vi "Do_Every_minute.vi"(1 "Ch Names":string[](array[string]), 2 "Values":dbl[](array[numeric]) format="%.2f") -> ()   [LabVIEW 2014]
uses:
  Do_Every_5mins.ctl
  Anemometry/Anemometry Sub Vis/Controls/In_Range.ctl
  ADAM Client/Sub VIs/ADAM Controls/Traverse_Level_State.ctl
  ADAM Client/Sub VIs/ADAM Controls/Valco_valve_ph.ctl
  <vilib>/Analysis/baseanly.llb/Mean (DBL).vi
  ADAM_Global.vi
  <vilib>/Analysis/NI_AALBase.lvlib
panel:
  in  "Disable Sending email to estates regarding Chilled water Temp":bool=TRUE
  in  "Max K Factor":dbl=2.7
  out "Case":T1
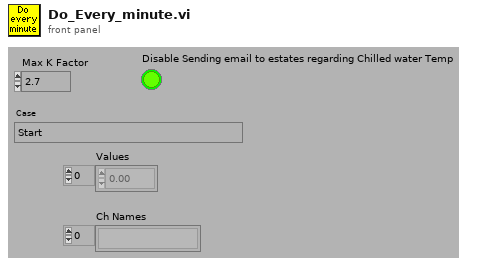
[diagram p1: front panel]
types:
  T1 = typedef "Do_Every_5mins.ctl" = enum16{"Start", "Update EnFlo Tunnel Speed Tweak", "Are EnFlo Tun Fan Bearings too Hot?", "Check EnFlo tweak factor?", "Are Inlet Screens Blocked?", "Tweak demanded chilled water temp", "Is Dew point meter Alive?", "Condensation Occurring", "Condensation Alert", "More checks", "Set FFID Valve to Measure", "End"}
  T2 = typedef "In_Range.ctl" = enum16{"%", "±", "% & ±"}
  T3 = typedef "Traverse_Level_State.ctl" = enum16{"Running", "Complete"}
  T4 = typedef "Client_State_Cluster.ctl" = cluster{"Client Name":string, "Traverse level State":T3, "People to Email":string[], "Next Contact Time":dbl}
  T5 = typedef "Valco_valve_ph.ctl" = u16
  T6 = cluster{"second":i32, "minute":i32, "hour":i32, "day of month":i32, "month":i32, "year":i32, "day of week":i32, "day of year":i32, "is DST":i32}
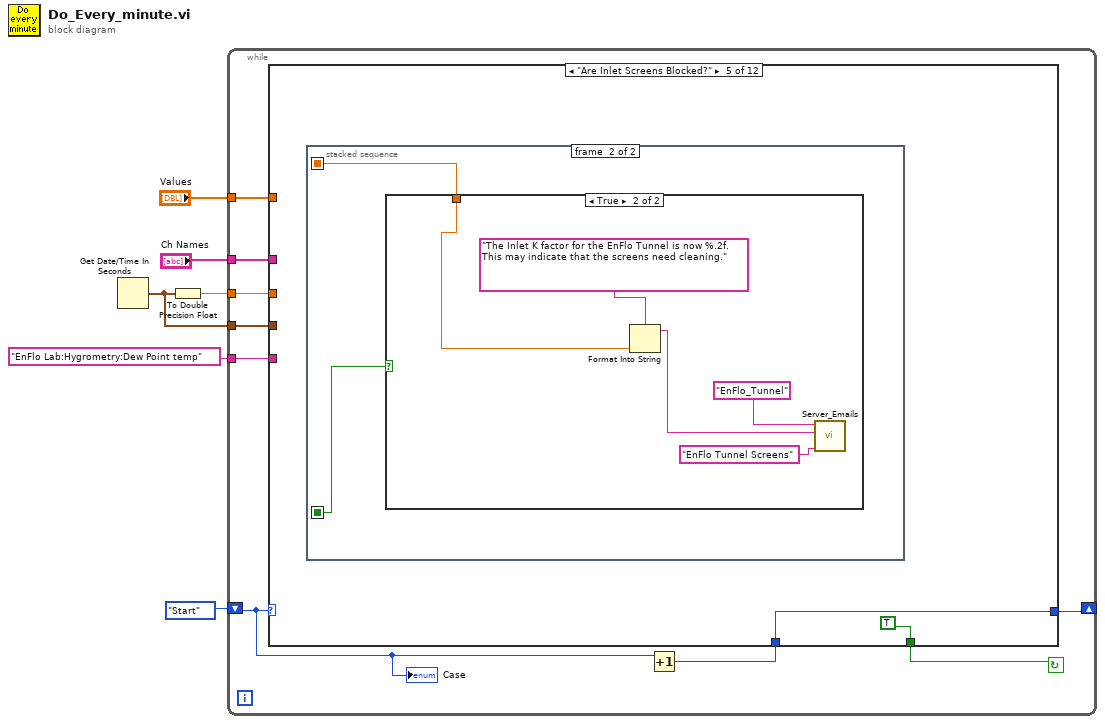
[diagram p0: block diagram]
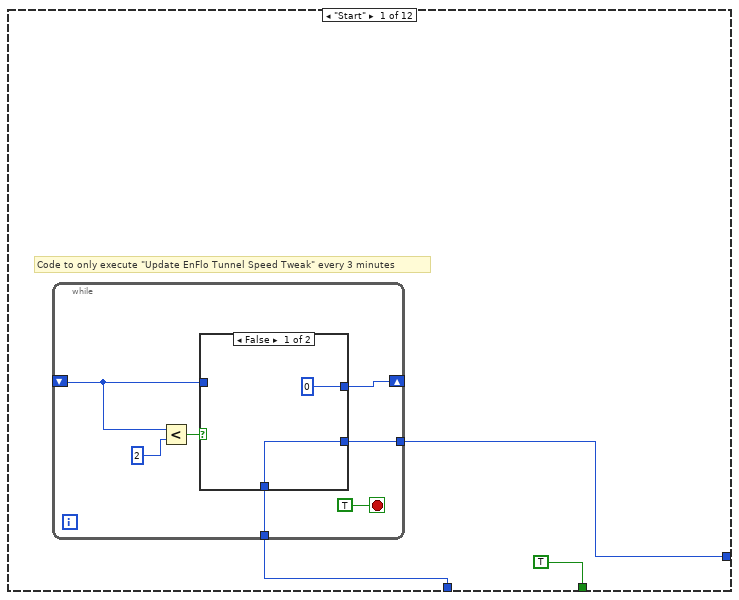
[diagram p2: hidden frame]
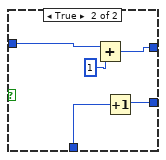
[diagram p3: hidden frame]
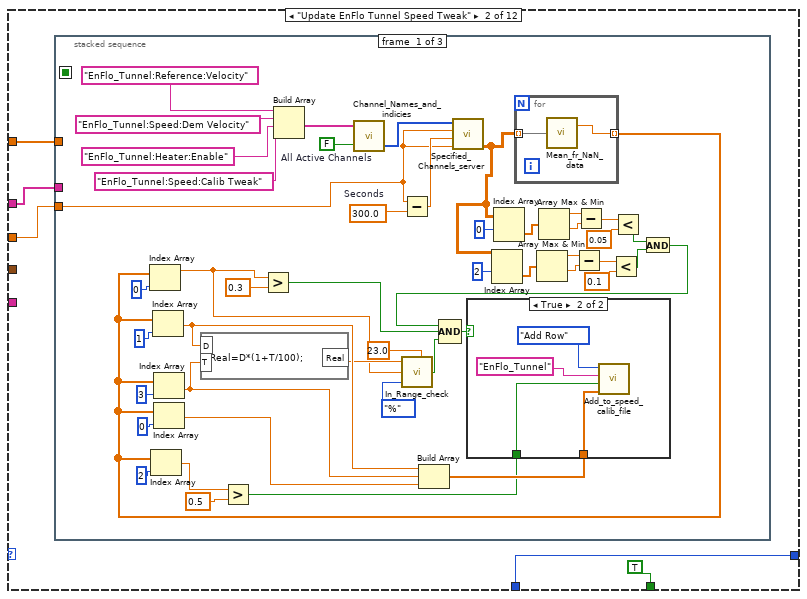
[diagram p4: hidden frame]
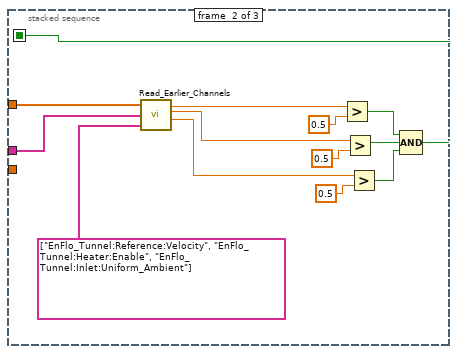
[diagram p6: hidden frame]
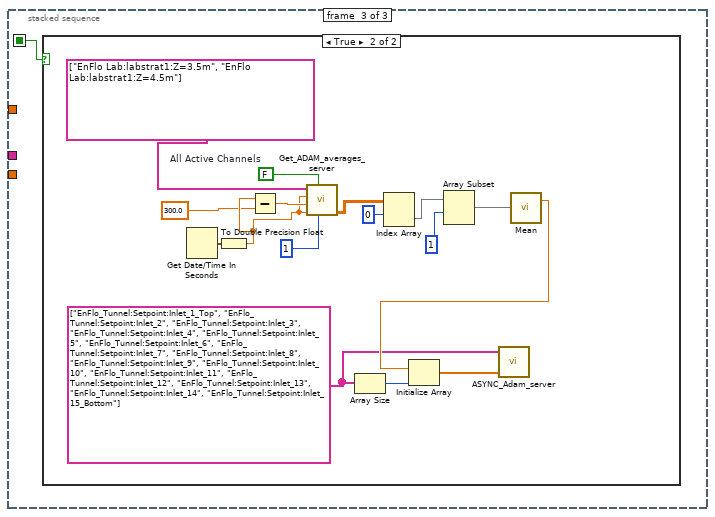
[diagram p7: hidden frame]
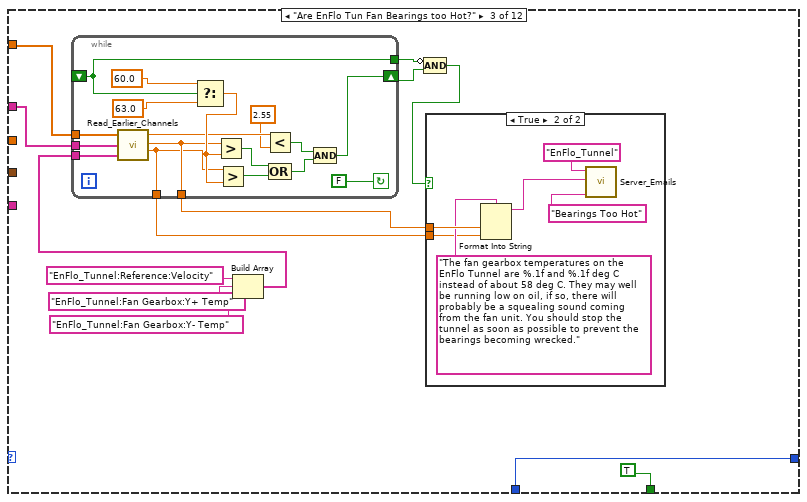
[diagram p9: hidden frame]
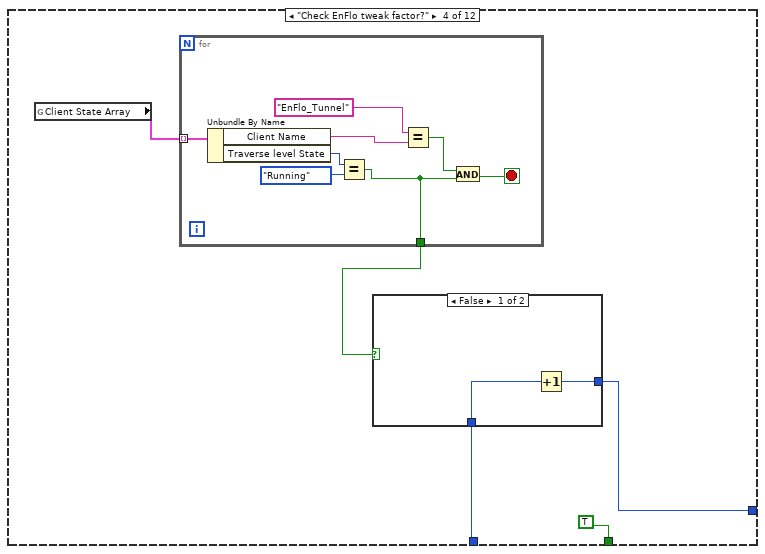
[diagram p11: hidden frame]
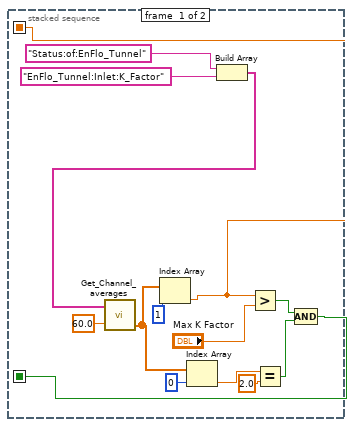
[diagram p13: hidden frame]
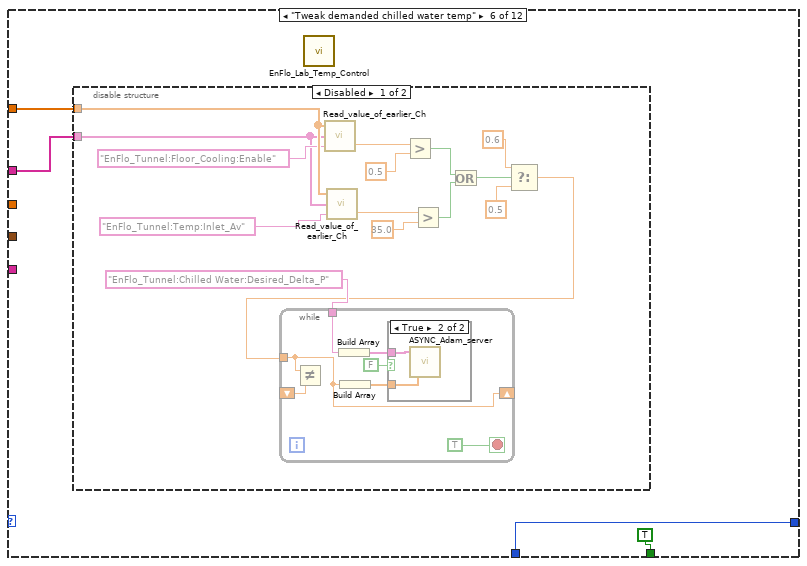
[diagram p15: hidden frame]
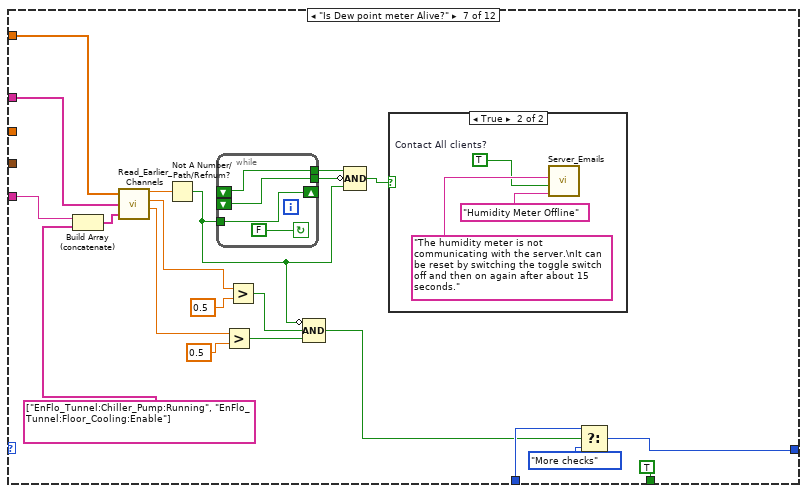
[diagram p18: hidden frame]
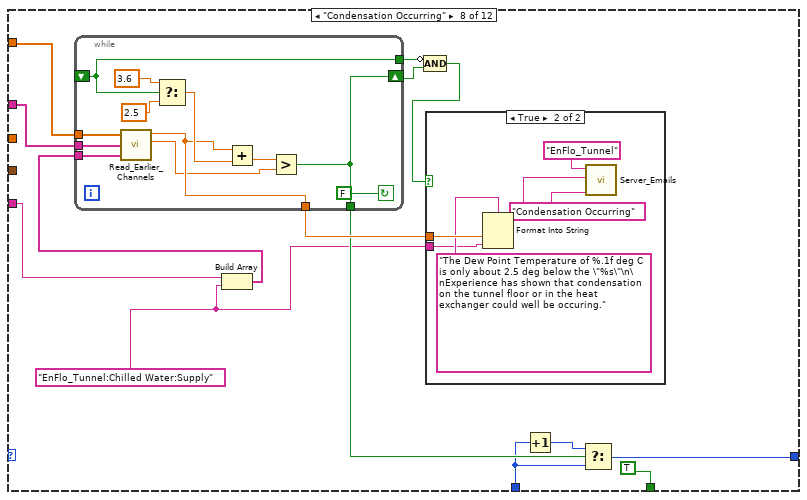
[diagram p20: hidden frame]
diagram:
  n1 = Get Date/Time In Seconds() -> (seconds since 1Jan1904=w1:timestamp)
  n2 = To Double Precision Float(number=w1) -> (double precision float=w2:dbl)
  n3 = while {
    tunnel: "EnFlo Lab:Hygrometry:Dew Point temp" -> [w9]
    tunnel: "Values" -> [w13]
    tunnel: "Ch Names" -> [w14]
    shift-left: Do_Every_5mins."Start" ("Case") -> [w10]
    shift-right: [w11] -> _
    tunnel: w2 -> [w8]
    tunnel: w1 -> [w7]
    stop <- w15 continue-if-true
    n4 = Increment(x=w10) -> (x+1=w12:T1)
    n5 = case shown="\"Are Inlet Screens Blocked?\"" w10 {
      tunnel: [TRUE TRUE TRUE TRUE TRUE TRUE TRUE TRUE TRUE TRUE TRUE FALSE] -> w15
      tunnel: w14 -> [_ w34 w130 _ _ w196 w240 w263 w290 w333 w342 w376]
      tunnel: w13 -> [_ w33 w131 _ _ w197 w241 w264 w291 w334 w341 w375]
      tunnel: w12 -> [w16 w37 w121 w159 w173 w199 w234 w254 w293 w331 w360 w379]
      tunnel: [w17 w37 w121 w158 w173 w199 w244 w255 w293 w330 w360 w379] -> w11
      tunnel: w9 -> [_ _ _ _ _ _ w239 w257 w284 _ _ _]
      tunnel: w8 -> [_ w35 _ _ _ _ _ _ _ _ w359 w374]
      tunnel: w7 -> [_ _ _ _ _ _ _ _ _ _ _ w377]
      frame "Start" {
        # "Code to only execute \"Update EnFlo Tunnel Speed Tweak\" every 3 minutes"
        n6 = while {
          shift-right: [w22] -> _
          shift-left: _ -> [w19]
          tunnel: [w21] -> w17
          tunnel: w16 -> [w20]
          stop <- TRUE stop-if-true
          n7 = Less?(x=w19, y=2) -> (x < y?=w23:bool)
          n8 = case shown="False" w23 {
            tunnel: [0 w30] -> w22
            tunnel: [w26 w28] -> w21
            tunnel: w20 -> [w26 w29]
            tunnel: w19 -> [_ w31]
            frame False {
            }
            frame True {
              n9 = Add(x=w31, y=1) -> (x+y=w30:i32)
              n10 = Increment(x=w29) -> (x+1=w28:T1)
            }
          }
        }
      }
      frame "Update EnFlo Tunnel Speed Tweak" {
        n11 = stacked-sequence {
          seq-local: [_ w91 _] -> [_ _ w104]
          tunnel: w35 -> [w38 _ _]
          tunnel: w34 -> [_ w103 _]
          tunnel: w33 -> [_ w102 _]
          frame #0 {
            w69 = 300.0  # Seconds
            w71 = FALSE  # All Active Channels
            n12 = Build Array("EnFlo_Tunnel:Reference:Velocity", "EnFlo_Tunnel:Speed:Dem Velocity", "EnFlo_Tunnel:Heater:Enable", "EnFlo_Tunnel:Speed:Calib Tweak") -> (w68:string[])
            n13 = call "Channel_Names_and_indicies.vi"("All Active Channels"=w71, "Desired Ch Names"=w68) -> ("Indicies"=w70:i32[])  [unwired: 1 out]
            n14 = Subtract(x=w38, y=w69) -> (x-y=w67:dbl)
            n15 = call "Specified_Channels_server.vi"("End time"=w38, "Start time"=w67, "Clients time"=w38, "Requested channels"=w70) -> ("Output array"=w49:dbl[][])  [unwired: 1 in, 4 out]
            n16 = Index Array(array=w49, index (row)=2 ("Index")) -> (element=w51:dbl[])  [unwired: 1 in]
            n17 = Index Array(array=w49, index (row)=0 ("Index")) -> (element=w65:dbl[])  [unwired: 1 in]
            n18 = for {
              tunnel: w49 -> [w86] mode=indexing
              tunnel: [w85] -> w58 mode=indexing
              n19 = call "Mean_fr_NaN_data.vi"("Data"=w86) -> ("Mean value"=w85:dbl)  [unwired: 1 out]
            }
            n20 = Index Array(array=w58, index=0) -> (element=w42:dbl)
            n21 = Index Array(array=w58, index=2) -> (element=w76:dbl)
            n22 = Index Array(array=w58, index=1) -> (element=w44:dbl)
            n23 = Index Array(array=w58, index=3) -> (element=w45:dbl)
            n24 = Index Array(array=w58, index=0) -> (element=w56:dbl)
            n25 = formula code="Real=D*(1+T/100);"("D"=w44, "T"=w45) -> ("Real"=w43:dbl)
            n26 = Greater?(x=w76, y=0.5) -> (0:w57:bool)
            n27 = Greater?(x=w42, y=0.3) -> (0:w74:bool)
            n28 = call "In_Range_check.vi"("%"=23.0, "Mode"=In_Range."%", "Value"=w42, "Setpoint"=w43) -> ("In Range"=w39:bool)  [unwired: 1 in, 2 out]
            n29 = Build Array(w44, w45, w56) -> (w73:dbl[])
            n30 = Array Max & Min(array=w51) -> (max value=w52:dbl, min value=w53:dbl)  [unwired: 2 out]
            n31 = Array Max & Min(array=w65) -> (max value=w64:dbl, min value=w63:dbl)  [unwired: 2 out]
            n32 = Subtract(x=w52, y=w53) -> (x-y=w54:dbl)
            n33 = Subtract(x=w64, y=w63) -> (x-y=w62:dbl)
            n34 = Less?(x=w54, y=0.1) -> (x < y?=w48:bool)
            n35 = Less?(x=w62, y=0.05) -> (x < y?=w47:bool)
            n36 = And(x=w47, y=w48) -> (x .and. y?=w46:bool)
            n37 = Compound Arithmetic op=AND(w46, w74, w39) -> (w72:bool)
            n38 = case shown="True" w72 {
              tunnel: w73 -> [_ w89]
              tunnel: w57 -> [_ w88]
              frame False {
              }
              frame True {
                n39 = call "Add_to_speed_calib_file.vi"("New Row"=w89, "Tunnel Heated?"=w88, "Rig Name"="EnFlo_Tunnel" ("y"), "Mode"=enum16{"Add Row", "Get Error Value"}."Add Row") -> ()  [unwired: 2 in, 2 out]
              }
            }
          }
          frame #1 {
            n40 = call "Read_Earlier_Channels.vi"("Present scan array"=w102, "Ch names"=w103, "Desired Channels"=string[] ["EnFlo_Tunnel:Reference:Velocity", "EnFlo_Tunnel:Heater:Enable", "EnFlo_Tunnel:Inlet:Uniform_Ambient"]) -> ("Index 0"=w100:dbl, "Index 1"=w96:dbl, "Index 2"=w95:dbl)  [unwired: 3 out]
            n41 = Greater?(x=w100, y=0.5) -> (0:w94:bool)
            n42 = Greater?(x=w96, y=0.5) -> (0:w93:bool)
            n43 = Greater?(x=w95, y=0.5) -> (0:w92:bool)
            n44 = Compound Arithmetic op=AND(w94, w93, w92) -> (w91:bool)
          }
          frame #2 {
            n45 = case shown="True" w104 {
              frame False {
              }
              frame True {
                w105 = string[] ["EnFlo_Tunnel:Setpoint:Inlet_1_Top", "EnFlo_Tunnel:Setpoint:Inlet_2", "EnFlo_Tunnel:Setpoint:Inlet_3", "EnFlo_Tunnel:Setpoint:Inlet_4", "EnFlo_Tunnel:Setpoint:Inlet_5", "EnFlo_Tunnel:Setpoint:Inlet_6", "EnFlo_Tunnel:Setpoint:Inlet_7", "EnFlo_Tunnel:Setpoint:Inlet_8", "EnFlo_Tunnel:Setpoint:Inlet_9", "EnFlo_Tunnel:Setpoint:Inlet_10", "EnFlo_Tunnel:Setpoint:Inlet_11", "EnFlo_Tunnel:Setpoint:Inlet_12", "EnFlo_Tunnel:Setpoint:Inlet_13", "EnFlo_Tunnel:Setpoint:Inlet_14", "EnFlo_Tunnel:Setpoint:Inlet_15_Bottom"] ("Desired Channels")
                w117 = FALSE  # All Active Channels
                n46 = Get Date/Time In Seconds() -> (seconds since 1Jan1904=w120:timestamp)
                n47 = To Double Precision Float(number=w120) -> (double precision float=w118:dbl)
                n48 = Subtract(x=w118, y=300.0) -> (x-y=w119:dbl)
                n49 = call "Get_ADAM_averages_server.vi"("No of averages"=1, "All Active Channels"=w117, "End time"=w118, "Start time"=w119, "Clients time"=w118, "ADAM Ch Names"=string[] ["EnFlo Lab:labstrat1:Z=3.5m", "EnFlo Lab:labstrat1:Z=4.5m"] ("Desired Channels")) -> ("DBL values"=w115:dbl[][])  [unwired: 4 out]
                n50 = Array Size(array=w105) -> (size(s)=w108:i32)
                n51 = Index Array(array=w115, index (row)=0) -> (element=w112:dbl[])  [unwired: 1 in]
                n52 = Array Subset(array=w112, index=1) -> (w109:dbl[])  [unwired: 1 in]
                n53 = call-poly <vilib>:"Mean.vi"("X"=w109) -> ("mean"=w107:dbl)  [unwired: 1 out]
                n54 = Initialize Array(w107, w108) -> (w106:dbl[])
                n55 = call "ASYNC_Adam_server.vi"("Values"=w106, "Channel Names"=w105) -> ()  [unwired: 1 in, 3 out]
              }
            }
          }
        }
      }
      frame "Are EnFlo Tun Fan Bearings too Hot?" {
        n56 = Build Array("EnFlo_Tunnel:Reference:Velocity", "EnFlo_Tunnel:Fan Gearbox:Y+ Temp", "EnFlo_Tunnel:Fan Gearbox:Y- Temp") -> (w129:string[])
        n57 = while {
          tunnel: [w135] -> w122
          tunnel: [w136] -> w123
          tunnel: [w145] -> w128
          shift-left: _ -> [w145]
          shift-right: [w137] -> w127
          tunnel: w129 -> [w148]
          tunnel: w130 -> [w149]
          tunnel: w131 -> [w150]
          stop <- FALSE continue-if-true
          n58 = call "Read_Earlier_Channels.vi"("Present scan array"=w150, "Ch names"=w149, "Desired Channels"=w148) -> ("Index 0"=w143:dbl, "Index 1"=w136:dbl, "Index 2"=w135:dbl)  [unwired: 3 out]
          n59 = Select(t=60.0, s=w145, f=63.0) -> (s? t:f=w144:dbl)
          n60 = Greater?(x=w136, y=w144) -> (0:w141:bool)
          n61 = Greater?(x=w135, y=w144) -> (0:w140:bool)
          n62 = Less?(x=w143, y=2.55) -> (x < y?=w139:bool)
          n63 = Compound Arithmetic op=OR(w141, w140) -> (w138:bool)
          n64 = Compound Arithmetic op=AND(w139, w138) -> (w137:bool)
        }
        n65 = Compound Arithmetic op=AND(invert w128, w127) -> (w126:bool)
        n66 = case shown="True" w126 {
          tunnel: w123 -> [_ w154]
          tunnel: w122 -> [_ w151]
          frame False {
          }
          frame True {
            n67 = Format Into String(format string="The fan gearbox temperatures on the EnFlo Tunnel are %.1f and %.1f deg C instead of about 58 deg C. They may well be running low on oil, if so, there will probably be a squealing sound coming from the fan unit. You should stop the tunnel as soon as possible to prevent the bearings becoming wrecked." ("Format String"), w154, w151) -> (resulting string=w153:string)  [unwired: 2 in, 1 out]
            n68 = call "Server_Emails.vi"("Client Name Contains"="EnFlo_Tunnel", "Message"=w153, "Subject"="Bearings Too Hot" ("Error Type")) -> ()  [unwired: 2 in, 3 out]
          }
        }
      }
      frame "Check EnFlo tweak factor?" {
        n69 = global read "ADAM_Global.vi" "Client State Array"() -> (w160:T4[])
        n70 = for {
          tunnel: w160 -> [w172] mode=indexing
          tunnel: [w165] -> w157
          stop <- w166 stop-if-true
          n71 = Unbundle By Name(w172) -> ("Client Name"=w168:string, "Traverse level State"=w171:T3)
          n72 = Equal?(x=w171, y=Traverse_Level_State."Running" ("Traverse level State")) -> (x = y?=w165:bool)
          n73 = Equal?(x="EnFlo_Tunnel" ("y"), y=w168) -> (x = y?=w167:bool)
          n74 = And(x=w167, y=w165) -> (x .and. y?=w166:bool)
        }
        n75 = case shown="False" w157 {
          tunnel: w159 -> [w163 w164]
          tunnel: [w162 w164] -> w158
          frame False {
            n76 = Increment(x=w163) -> (x+1=w162:T1)
          }
          frame True {
          }
        }
      }
      frame "Are Inlet Screens Blocked?" {
        n77 = stacked-sequence {
          seq-local: [w175 _] -> [_ w190]
          seq-local: [w178 _] -> [_ w189]
          frame #0 {
            n78 = Build Array("Status:of:EnFlo_Tunnel", "EnFlo_Tunnel:Inlet:K_Factor") -> (w180:string[])
            n79 = call "Get_Channel_averages.vi"("Desired Ch Names"=w180, "Averaging time (mins)"=60.0) -> ("number"=w186:dbl[])  [unwired: 1 in, 2 out]
            n80 = Index Array(array=w186, index=1) -> (element=w175:dbl)
            n81 = Index Array(array=w186, index=0) -> (element=w185:dbl)
            n82 = Greater?(x=w175, y="Max K Factor") -> (0:w177:bool)
            n83 = Equal?(x=w185, y=2.0) -> (x = y?=w183:bool)
            n84 = Compound Arithmetic op=AND(w177, w183) -> (w178:bool)
          }
          frame #1 {
            n85 = case shown="True" w189 {
              tunnel: w190 -> [_ w194]
              frame False {
              }
              frame True {
                n86 = Format Into String(format string="The Inlet K factor for the EnFlo Tunnel is now %.2f. This may indicate that the screens need cleaning." ("Format String"), w194) -> (resulting string=w192:string)  [unwired: 2 in, 1 out]
                n87 = call "Server_Emails.vi"("Client Name Contains"="EnFlo_Tunnel", "Message"=w192, "Subject"="EnFlo Tunnel Screens" ("Message")) -> ()  [unwired: 2 in, 3 out]
              }
            }
          }
        }
      }
      frame "Tweak demanded chilled water temp" {
        n88 = disable-structure shown="Disabled" {
          disable-tunnel: w197 -> [w213 _]
          disable-tunnel: w196 -> [w211 _]
          frame Disabled {
            n89 = call "Read_value_of_earlier_Ch.vi"("Desired Ch to Read"="EnFlo_Tunnel:Floor_Cooling:Enable", "Ch names"=w211, "Present scan array"=w213) -> ("Value"=w209:dbl)  [unwired: 1 in, 1 out]
            n90 = call "Read_value_of_earlier_Ch.vi"("Desired Ch to Read"="EnFlo_Tunnel:Temp:Inlet_Av", "Ch names"=w211, "Present scan array"=w213) -> ("Value"=w207:dbl)  [unwired: 1 in, 1 out]
            n91 = Greater?(x=w209, y=0.5) -> (0:w205:bool)
            n92 = Greater?(x=w207, y=35.0) -> (0:w204:bool)
            n93 = Or(x=w205, y=w204) -> (x .or. y?=w203:bool)
            n94 = Select(t=0.6, s=w203, f=0.5 ("t")) -> (s? t:f=w200:dbl)
            n95 = while {
              shift-right: [w217] -> _
              shift-left: _ -> [w218]
              tunnel: w200 -> [w217]
              tunnel: "EnFlo_Tunnel:Chilled Water:Desired_Delta_P" -> [w219]
              stop <- TRUE stop-if-true
              n96 = Not Equal?(x=w217, y=w218) -> ()  [unwired: 1 out]
              n97 = Build Array(w219) -> (w220:string[])
              n98 = Build Array(w217) -> (w221:dbl[])
              n99 = case shown="True" FALSE {
                tunnel: w221 -> [_ w223]
                tunnel: w220 -> [_ w222]
                frame False {
                }
                frame True {
                  n100 = call "ASYNC_Adam_server.vi"("Values"=w223, "Channel Names"=w222) -> ()  [unwired: 1 in, 3 out]
                }
              }
            }
          }
          frame Enabled {
          }
        }
        n101 = call "EnFlo_Lab_Temp_Control.vi"() -> ()  [unwired: 1 out]
      }
      frame "Is Dew point meter Alive?" {
        n102 = Build Array (concatenate)(w239, string[] ["EnFlo_Tunnel:Chiller_Pump:Running", "EnFlo_Tunnel:Floor_Cooling:Enable"] ("appended array")) -> (w238:string[])
        n103 = call "Read_Earlier_Channels.vi"("Present scan array"=w241, "Ch names"=w240, "Desired Channels"=w238) -> ("Index 0"=w237:dbl, "Index 1"=w236:dbl, "Index 2"=w225:dbl)  [unwired: 3 out]
        n104 = Not A Number/Path/Refnum?(number/path/refnum=w237) -> (NaN/Path/Refnum?=w231:bool)
        n105 = while {
          tunnel: [w246] -> w229
          tunnel: [w247] -> w230
          shift-left: _ -> [w247]
          tunnel: w231 -> [w248]
          shift-left: _ -> [w246]
          shift-right: [w248] -> _
          stop <- FALSE continue-if-true
        }
        n106 = Greater?(x=w225, y=0.5) -> (0:w224:bool)
        n107 = Greater?(x=w236, y=0.5) -> (0:w235:bool)
        n108 = Compound Arithmetic op=AND(invert w231, w235, w224) -> (w232:bool)
        n109 = Compound Arithmetic op=AND(w229, invert w230, w231) -> (w242:bool)
        n110 = case shown="True" w242 {
          frame False {
          }
          frame True {
            w249 = TRUE  # Contact All clients?
            n111 = call "Server_Emails.vi"("Message"="The humidity meter is not communicating with the server.\nIt can be reset by switching the toggle switch off and then on again after about 15 seconds." ("Bundle Element"), "Contact All clients?"=w249, "Subject"="Humidity Meter Offline" ("Error Type")) -> ()  [unwired: 2 in, 3 out]
          }
        }
        n112 = Select(t=w234, s=w232, f=Do_Every_5mins."More checks" ("Case")) -> (s? t:f=w244:T1)
      }
      frame "Condensation Occurring" {
        w252 = "EnFlo_Tunnel:Chilled Water:Supply"
        n113 = Build Array(w257, w252) -> (w262:string[])
        n114 = while {
          tunnel: [w267] -> w256
          tunnel: [w269] -> w258
          tunnel: [w270] -> w261
          shift-left: _ -> [w270]
          shift-right: [w267] -> w260
          tunnel: w262 -> [w275]
          tunnel: w263 -> [w276]
          tunnel: w264 -> [w277]
          stop <- FALSE continue-if-true
          n115 = call "Read_Earlier_Channels.vi"("Present scan array"=w277, "Ch names"=w276, "Desired Channels"=w275) -> ("Index 0"=w269:dbl, "Index 1"=w268:dbl)  [unwired: 4 out]
          n116 = Select(t=3.6, s=w270, f=2.5) -> (s? t:f=w271:dbl)
          n117 = Add(x=w269, y=w271) -> (x+y=w274:dbl)
          n118 = Greater?(x=w274, y=w268) -> (0:w267:bool)
        }
        n119 = Compound Arithmetic op=AND(invert w261, w260) -> (w259:bool)
        n120 = case shown="True" w259 {
          tunnel: w258 -> [_ w281]
          tunnel: w252 -> [_ w278]
          frame False {
          }
          frame True {
            n121 = Format Into String(format string="The Dew Point Temperature of %.1f deg C is only about 2.5 deg below the \"%s\"\n\nExperience has shown that condensation on the tunnel floor or in the heat exchanger could well be occuring." ("Format String"), w281, w278) -> (resulting string=w280:string)  [unwired: 2 in, 1 out]
            n122 = call "Server_Emails.vi"("Client Name Contains"="EnFlo_Tunnel", "Message"=w280, "Subject"="Condensation Occurring" ("Error Type")) -> ()  [unwired: 2 in, 3 out]
          }
        }
        n123 = Increment(x=w254) -> (x+1=w253:T1)
        n124 = Select(t=w253, s=w256, f=w254) -> (s? t:f=w255:T1)
      }
      frame "Condensation Alert" {
        n125 = Build Array(w284, "EnFlo_Tunnel:Chilled Water:Dem Temp") -> (w289:string[])
        n126 = while {
          tunnel: [w297] -> w285
          tunnel: [w299] -> w288
          shift-left: _ -> [w299]
          shift-right: [w298] -> w287
          tunnel: w289 -> [w304]
          tunnel: w290 -> [w305]
          tunnel: w291 -> [w306]
          stop <- FALSE continue-if-true
          n127 = call "Read_Earlier_Channels.vi"("Present scan array"=w306, "Ch names"=w305, "Desired Channels"=w304) -> ("Index 0"=w297:dbl, "Index 1"=w296:dbl)  [unwired: 4 out]
          n128 = Select(t=4.0, s=w299, f=3.5) -> (s? t:f=w300:dbl)
          n129 = Add(x=w297, y=w300) -> (x+y=w303:dbl)
          n130 = Greater?(x=w303, y=w296) -> (0:w298:bool)
        }
        n131 = Compound Arithmetic op=AND(invert w288, w287) -> (w286:bool)
        n132 = case shown="True" w286 {
          tunnel: w285 -> [_ w309]
          frame False {
          }
          frame True {
            n133 = Format Into String(format string="The Dew Point Temperature is only about 3.5 degrees below the chilled water setpoint temperature.\n\nExperience has shown that unless the chilled water setpoint temperature is adjusted, condensation on the tunnel floor will occur if the dew point temperature (currently at %.1f degrees) rises by much more than one degree." ("Format String"), w309) -> (resulting string=w308:string)  [unwired: 2 in, 1 out]
            n134 = call "Server_Emails.vi"("Client Name Contains"="EnFlo_Tunnel", "Message"=w308, "Subject"="Condensation Alert" ("Error Type")) -> ()  [unwired: 2 in, 3 out]
          }
        }
      }
      frame "More checks" {
        w313 = "EnFlo_Tunnel:Extra_Lights:Enable"
        n135 = Build Array("Fast FID:Valco Valve:Position", "Status:of:EnFlo_Tunnel", w313) -> (w328:string[])
        n136 = call "Read_Earlier_Channels.vi"("Present scan array"=w334, "Ch names"=w333, "Desired Channels"=w328) -> ("Index 0"=w321:dbl, "Index 1"=w319:dbl, "Index 2"=w317:dbl)  [unwired: 3 out]
        n137 = Greater?(x=w317, y=0.5) -> (0:w315:bool)
        n138 = Equal?(x=w319, y=2.0) -> (x = y?=w314:bool)
        n139 = And(x=w314, y=w315) -> (x .and. y?=w312:bool)
        n140 = disable-structure shown="Disabled" {
          disable-tunnel: w313 -> [w337 _]
          disable-tunnel: w312 -> [w336 _]
          frame Disabled {
            n141 = case shown="True" w336 {
              tunnel: w337 -> [_ w340]
              frame False {
              }
              frame True {
                n142 = Build Array(w340) -> (w339:string[])
                n143 = call "ASYNC_Adam_server.vi"("Values"=dbl[] [0.0], "Channel Names"=w339) -> ()  [unwired: 1 in, 3 out]
              }
            }
          }
          frame Enabled {
          }
        }
        n144 = Equal?(x=4.0, y=w321) -> (x = y?=w325:bool)
        n145 = Equal?(x=1.0, y=w321) -> (x = y?=w324:bool)
        n146 = Not A Number/Path/Refnum?(number/path/refnum=w321) -> (NaN/Path/Refnum?=w326:bool)
        n147 = Compound Arithmetic op=OR(w324, w325, w326) -> (w323:bool)
        n148 = Select(t=Do_Every_5mins."End" ("Case"), s=w323, f=w331) -> (s? t:f=w330:T1)
      }
      frame "Set FFID Valve to Measure" {
        w358 = FALSE  # All Active Channels
        n149 = Build Array("Fast FID:Valco Valve:Position") -> (w356:string[])
        n150 = call "Channel_Names_and_indicies.vi"("All Active Channels"=w358, "Desired Ch Names"=w356) -> ("Indicies"=w357:i32[])  [unwired: 1 out]
        n151 = Subtract(x=w359, y=700.0) -> (x-y=w354:dbl)
        n152 = call "Specified_Channels_server.vi"("End time"=w359, "Start time"=w354, "Clients time"=w359, "Requested channels"=w357) -> ("Output array"=w351:dbl[][])  [unwired: 1 in, 4 out]
        n153 = Index Array(array=w351, index (row)=0 ("Index")) -> (element=w347:dbl[])  [unwired: 1 in]
        n154 = Not A Number/Path/Refnum?(number/path/refnum=w347) -> (NaN/Path/Refnum?=w346:bool[])
        n155 = Or Array Elements(Boolean array=w346) -> (logical OR=w344:bool)
        n156 = Array Max & Min(array=w347) -> (max value=w349:dbl, min value=w350:dbl)  [unwired: 2 out]
        n157 = Subtract(x=w349, y=w350) -> (x-y=w348:dbl)
        n158 = Equal To 0?(x=w348) -> (x = 0?=w345:bool)
        n159 = Compound Arithmetic op=AND(w345, invert w344) -> (w343:bool)
        n160 = case shown="True" w343 {
          tunnel: w342 -> [_ w368]
          tunnel: w341 -> [_ w367]
          frame False {
          }
          frame True {
            n161 = Build Array("FFID:System:Enable") -> (w365:string[])
            n162 = call "Read_Earlier_Channels.vi"("Present scan array"=w367, "Ch names"=w368, "Desired Channels"=w365) -> ("Index 0"=w364:dbl)  [unwired: 5 out]
            n163 = Greater?(x=w364, y=0.5) -> (0:w362:bool)
            n164 = case shown="True" w362 {
              frame False {
                n165 = Build Array(0.0) -> (w369:dbl[])
                n166 = Build Array("GMU:Gas:Enable") -> (w370:string[])
                n167 = call "ASYNC_Adam_server.vi"("Values"=w369, "Channel Names"=w370) -> ()  [unwired: 1 in, 3 out]
              }
              frame True {
                w373 = T5 4 items=["", "Zero Air", "Calib 1", "Calib 2", "Measure"] ("Requested Position")
                n168 = call "Fast_FID_Valve_Control.vi"("Requested Position"=w373) -> ()  [unwired: 7 out]
              }
            }
          }
        }
      }
      frame "End" {
        n169 = stacked-sequence {
          seq-local: [w386 _ _] -> [_ w406 _]
          seq-local: [w380 _ _] -> [_ w403 _]
          tunnel: w377 -> [w391 _ _]
          tunnel: w376 -> [w383 w405 w422]
          tunnel: w375 -> [w384 w404 w423]
          tunnel: w374 -> [_ _ w418]
          frame #0 {
            n170 = call <vilib>:"LV70TimeStampToDateRec.vi"("time stamp"=w391) -> ("date time rec"=w392:T6)
            n171 = Unbundle By Name(w392) -> ("hour"=w390:i32, "day of week"=w389:i32)
            n172 = while {
              tunnel: w390 -> [w402]
              tunnel: w389 -> [w400]
              shift-right: [w395] -> w387
              shift-left: _ -> [w394]
              tunnel: [w394] -> w388
              stop <- FALSE continue-if-true
              n173 = Equal?(x=w402, y=10) -> (x = y?=w396:bool)
              n174 = In Range and Coerce(upper limit=7, x=w400, lower limit=1) -> (In Range?=w397:bool)  [unwired: 1 out]
              n175 = And(x=w396, y=w397) -> (x .and. y?=w395:bool)
            }
            n176 = call "Read_value_of_earlier_Ch.vi"("Desired Ch to Read"="Uni:Chilled Water:Temp", "Ch names"=w383, "Present scan array"=w384) -> ("Value"=w380:dbl)  [unwired: 1 in, 1 out]
            n177 = Greater?(x=w380, y=15.0) -> (0:w381:bool)
            n178 = Compound Arithmetic op=AND(w381, invert w388, w387) -> (w386:bool)
          }
          frame #1 {
            n179 = case shown="True" w406 {
              tunnel: w405 -> [_ _]
              tunnel: w404 -> [_ _]
              tunnel: w403 -> [_ w414]
              frame False {
              }
              frame True {
                n180 = Select(t=string[] [], s="Disable Sending email to estates regarding Chilled water Temp", f=string[] ["efmenquiries@surrey.ac.uk"] ("Extra People to Email")) -> (s? t:f=w407:string[])
                n181 = Format Into String(format string="Dear Estates\n\nThe monitoring system in the EnFlo Lab (01AB01) is currently indicating that the Chilled water in the AB Building is at %d deg C.\n\nPlease could you arrange for somebody to come and investigate this please.\n\nThanks very much\n\nPaul Hayden x9545  or Mobile  07961 608409", w414) -> (resulting string=w413:string)  [unwired: 2 in, 1 out]
                n182 = call "Server_Emails.vi"("Message"=w413, "Contact All clients?"=TRUE, "Subject"="Chilled water in AB Building above 15 deg C" ("Error Type"), "Extra People to Email"=w407) -> ()  [unwired: 1 in, 3 out]
              }
            }
          }
          frame #2 {
            w416 = "Aero_Tunnel:Seeder:Enable" ("Desired Ch to Read")
            n183 = call "Read_value_of_earlier_Ch.vi"("Desired Ch to Read"=w416, "Ch names"=w422, "Present scan array"=w423) -> ("Value"=w421:dbl)  [unwired: 1 in, 1 out]
            n184 = Greater?(x=w421, y=0.5) -> (0:w419:bool)
            n185 = case shown="True" w419 {
              tunnel: w416 -> [_ w433]
              tunnel: w418 -> [_ w432]
              tunnel: [FALSE w428] -> w417
              frame False {
              }
              frame True {
                w440 = FALSE  # All Active Channels
                n186 = Build Array(w433) -> (w438:string[])
                n187 = call "Channel_Names_and_indicies.vi"("All Active Channels"=w440, "Desired Ch Names"=w438) -> ("Indicies"=w439:i32[])  [unwired: 1 out]
                n188 = Subtract(x=w432, y=30.0) -> (x-y=w436:dbl)
                n189 = call "Specified_Channels_server.vi"("End time"=w432, "Start time"=w436, "Clients time"=w432, "Requested channels"=w439) -> ("Output array"=w434:dbl[][])  [unwired: 1 in, 4 out]
                n190 = Index Array(array=w434, index (row)=0 ("Index")) -> (element=w430:dbl[])  [unwired: 1 in]
                n191 = Greater?(x=w430, y=0.5) -> (0:w429:bool[])
                n192 = And Array Elements(Boolean array=w429) -> (logical AND=w428:bool)
              }
            }
            n193 = case shown="True" w417 {
              tunnel: w416 -> [_ w426]
              frame False {
              }
              frame True {
                n194 = Build Array(w426) -> (w425:string[])
                n195 = call "ASYNC_Adam_server.vi"("Values"=dbl[] [0.0], "Channel Names"=w425) -> ()  [unwired: 1 in, 3 out]
              }
            }
          }
        }
      }
    }
    "Case" <- w10
  }
